vi "FindMaximum_MotorPower.vi"() -> ()   [LabVIEW 2017]
uses:
  <vilib>/myRIO/Instrument Drivers/Onboard IO/DIO/typedefs/DIO Reference.ctl
  <vilib>/myRIO/Common/Instrument Driver Framework/Utilities/typedefs/myRIO Generic Hardware Reference.ctl
  <vilib>/myRIO/Common/Instrument Driver Framework/Utilities/typedefs/Hardware Version Enum.ctl
  <vilib>/myRIO/Common/Instrument Driver Framework/Utilities/typedefs/myRIO v1.0 Reference.ctl
  <vilib>/myRIO/Common/Instrument Driver Framework/Utilities/typedefs/Generic FPGA Reference.ctl
  <vilib>/myRIO/Common/Instrument Driver Framework/myRIO v1.0/DIO/typedefs/DIO Channels List.ctl
  <vilib>/myRIO/Common/Instrument Driver Framework/myRIO v1.0/DIO/typedefs/DIO Channels Enum.ctl
  <vilib>/userdefined/High Color/nirio_resource_hc.ctl
  <vilib>/myRIO/Common/Instrument Driver Framework/Utilities/vis/Is FPGA Ref Available.vi
  <vilib>/myRIO/Common/Instrument Driver Framework/myRIO v1.0/DIO/vis/myRIO v1.1 Open DIO.vi
  <vilib>/myRIO/Instrument Drivers/Onboard IO/DIO/vis/Read.vi
  <vilib>/myRIO/Common/Instrument Driver Framework/Utilities/vis/Validate Channels.vi
  <vilib>/myRIO/Common/Instrument Driver Framework/myRIO v1.0/DIO/vis/myRIO v1.0 Reserve DIO.vi
  <vilib>/myRIO/Common/Instrument Driver Framework/myRIO v1.0/UART/vis/myRIO v1.0 Close UART.vi
  <vilib>/myRIO/Common/Instrument Driver Framework/myRIO v1.0/Resource Manager/vis/myRIO v1.0 Reserve Channel List.vi
  <vilib>/myRIO/Common/Instrument Driver Framework/myRIO v1.0/DIO/vis/myRIO v1.0 Build MUX Configuration DIO.vi
  <vilib>/myRIO/Common/Instrument Driver Framework/myRIO v1.0/Resource Manager/vis/myRIO v1.0 Reserve Channel.vi
  <vilib>/myRIO/Common/Instrument Driver Framework/myRIO v1.0/Resource Manager/vis/myRIO v1.0 Unreserve Channel.vi
  <vilib>/myRIO/Common/Instrument Driver Framework/myRIO v1.0/Resource Manager/vis/myRIO v1.0 Create Configuration List.vi
  <vilib>/myRIO/Common/Instrument Driver Framework/myRIO v1.0/Resource Manager/vis/myRIO v1.0 Build Mutex Name.vi
  <vilib>/Utility/VariantDataType/GetNumericInfo.vi
  <vilib>/Utility/error.llb/Error Cluster From Error Code.vi
  <vilib>/myRIO/Common/Instrument Driver Framework/myRIO v1.0/myRIO v1.1 Open.vi
  <vilib>/myRIO/Common/Instrument Driver Framework/Utilities/vis/IO Manager.vi
  <vilib>/myRIO/Common/Instrument Driver Framework/Utilities/vis/Configuration Manager.vi
  <vilib>/myRIO/Common/Instrument Driver Framework/myRIO v1.0/Resource Manager/vis/myRIO v1.0 Configure IO.vi
  <vilib>/myRIO/Common/Instrument Driver Framework/myRIO v1.0/myRIO v1.0 Close.vi
  <vilib>/myRIO/Common/Instrument Driver Framework/myRIO v1.0/DIO/vis/myRIO v1.0 Read DIO.vi
  <vilib>/myRIO/Common/Instrument Driver Framework/Utilities/vis/FPGA Ref Manager.vi
  <vilib>/myRIO/Common/Instrument Driver Framework/myRIO v1.0/myRIO v1.0 Reset FPGA.vi
  <vilib>/myRIO/Common/Instrument Driver Framework/myRIO v1.0/IRQ/vis/myRIO v1.0 IRQ Info FGV.vi
  <vilib>/myRIO/Common/Instrument Driver Framework/myRIO v1.0/IRQ/vis/myRIO v1.0 Timer IRQ Info FGV.vi
  <vilib>/myRIO/Common/Instrument Driver Framework/myRIO v1.0/IRQ/vis/myRIO v1.0 ISR Agent.vi
  <vilib>/myRIO/Express VI/Onboard Devices/Button/Button Express VI.xnode
  <vilib>/myRIO/Instrument Drivers/Onboard IO/DIO/vis/myRIO DIO Open.xnode
  <vilib>/myRIO/Instrument Drivers/Onboard IO/DIO/DIO.lvlib
  <vilib>/myRIO/Instrument Drivers/Utilities/Utilities.lvlib
panel:
  out "error out":errorcluster
  in  "milliseconds to wait":u32=3000
  in  "w2":i8(slide)=-100 scale=-100.0..100.0
  in  "w1":i8(slide)=-100 scale=-100.0..100.0
  in  "w3":i8(slide)=100 scale=-100.0..100.0
  in  "w4":i8(slide)=100 scale=-100.0..100.0
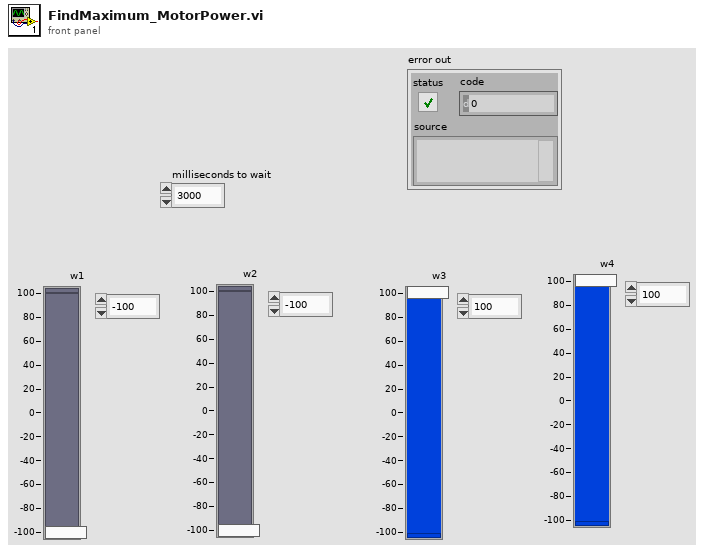
[diagram p1: front panel]
types:
  T1 = typedef "DIO.lvlib/DIO Reference.ctl" = cluster{"myRIO Reference":T2, "DIO Channels List":T6}
  T2 = typedef "myRIO Generic Hardware Reference.ctl" = cluster{"myRIO Model":T3, "myRIO Hardware Reference":T4}
  T3 = typedef "Hardware Version Enum.ctl" = enum16{"Unknown", "myRIO-1900", "myRIO-1950", "roboRIO", "NI ELVIS RIO CM"}
  T4 = typedef "myRIO v1.0 Reference.ctl" = cluster{"Generic FPGA Reference":T5, "Allow multiple opens":bool}
  T5 = typedef "Generic FPGA Reference.ctl" = refnum<k20>
  T6 = typedef "DIO Channels List.ctl" = T7[]
  T7 = typedef "DIO Channels Enum.ctl" = enum16{"Not Connected", "C/DIO0", "C/DIO1", "C/DIO2", "C/DIO3", "C/DIO4", "C/DIO5", "C/DIO6", "C/DIO7", "A/DIO0", "A/DIO1", "A/DIO2", "A/DIO3", "A/DIO4", "A/DIO5", "A/DIO6", "A/DIO7", "A/DIO8", "A/DIO9", "A/DIO10", "A/DIO11", "A/DIO12", "A/DIO13", "A/DIO14", "A/DIO15", "B/DIO0", "B/DIO1", "B/DIO2", "B/DIO3", "B/DIO4", "B/DIO5", "B/DIO6", "B/DIO7", "B/DIO8", "B/DIO9", "B/DIO10", "B/DIO11", "B/DIO12", "B/DIO13", "B/DIO14", "B/DIO15", "LED0", "LED1", "LED2", "LED3", "Button0", "DIO/DIO0", "DIO/DIO1", "DIO/DIO2", "DIO/DIO3", "DIO/DIO4", "DIO/DIO5", "DIO/DIO6", "DIO/DIO7", "DIO/DIO8", "DIO/DIO9", "SPI/CS0", "SPI/CS1", "SPI/CS2", "SPI/CS3", "LED RADIO (Green)", "LED RADIO (Red)", "LED COMM (Green)", "LED COMM (Red)", "LED MODE (Green)", "LED MODE (Red)"}
  T8 = typedef "nirio_resource_hc.ctl" = tag
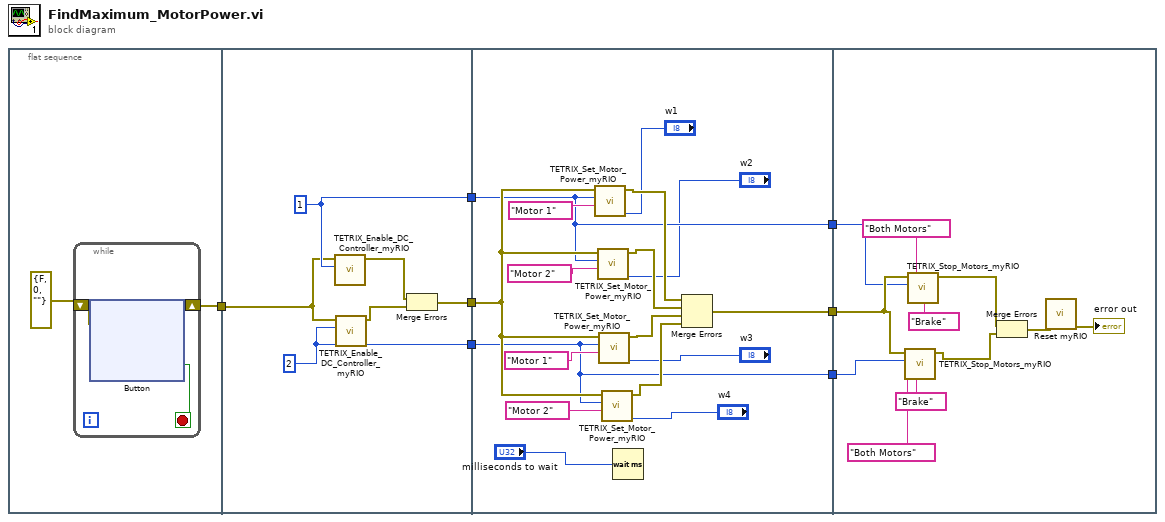
[diagram p0: block diagram]
diagram:
  n1 = flat-sequence {
    tunnel: [w9] -> w7
    tunnel: [w51] -> w6
    tunnel: [w50] -> w5
    tunnel: [w49] -> w4
    tunnel: w7 -> [w48]
    tunnel: w6 -> [w59]
    tunnel: w5 -> [w70]
    tunnel: w4 -> [w58]
    tunnel: [w61] -> w3
    tunnel: [w59] -> w2
    tunnel: [w58] -> w1
    tunnel: w3 -> [w81]
    tunnel: w2 -> [w80]
    tunnel: w1 -> [w79]
    frame #0 {
      n2 = while {
        shift-right: [w12] -> w9
        shift-left: errorcluster {"status"=FALSE, "code"=0, "source"=""} ("error constant") -> [w11]
        stop <- w10 stop-if-true
        n3 = xnode "Button"("error in (no error)"=w11) -> ("Value"=w10:bool, "error out"=w12:errorcluster)
      }
    }
    frame #1 {
      w49 = u8 2 ("Controller ID#  (I2C Address)")
      w51 = u8 1 ("Controller ID#  (I2C Address)")
      n4 = call <vilib>:"TETRIX_Enable_DC_Controller_myRIO.vi"("Controller ID#  (I2C Address)"=w51, "Error/Flow In"=w48) -> ("Error/Flow Out"=w53:errorcluster)  [unwired: 5 in]
      n5 = call <vilib>:"TETRIX_Enable_DC_Controller_myRIO.vi"("Controller ID#  (I2C Address)"=w49, "Error/Flow In"=w48) -> ("Error/Flow Out"=w52:errorcluster)  [unwired: 5 in]
      n6 = Merge Errors(w53, w52) -> (w50:errorcluster)
    }
    frame #2 {
      n7 = call <vilib>:"TETRIX_Set_Motor_Power_myRIO.vi"("Power (-100 to 100)  0 = Coast Stop  125 = Brake Stop"="w1", "Select Channel"="Motor 1", "Controller ID#  (I2C Address)"=w59, "Error/Flow In"=w70) -> ("Error/Flow Out"=w65:errorcluster)  [unwired: 3 in]
      n8 = call <vilib>:"TETRIX_Set_Motor_Power_myRIO.vi"("Power (-100 to 100)  0 = Coast Stop  125 = Brake Stop"="w2", "Select Channel"="Motor 2", "Controller ID#  (I2C Address)"=w59, "Error/Flow In"=w70) -> ("Error/Flow Out"=w64:errorcluster)  [unwired: 3 in]
      n9 = call <vilib>:"TETRIX_Set_Motor_Power_myRIO.vi"("Power (-100 to 100)  0 = Coast Stop  125 = Brake Stop"="w3", "Select Channel"="Motor 1", "Controller ID#  (I2C Address)"=w58, "Error/Flow In"=w70) -> ("Error/Flow Out"=w63:errorcluster)  [unwired: 3 in]
      n10 = call <vilib>:"TETRIX_Set_Motor_Power_myRIO.vi"("Power (-100 to 100)  0 = Coast Stop  125 = Brake Stop"="w4", "Select Channel"="Motor 2", "Controller ID#  (I2C Address)"=w58, "Error/Flow In"=w70) -> ("Error/Flow Out"=w62:errorcluster)  [unwired: 3 in]
      n11 = Wait (ms)(milliseconds to wait="milliseconds to wait") -> ()  [unwired: 1 out]
      n12 = Merge Errors(w65, w64, w63, w62) -> (w61:errorcluster)
    }
    frame #3 {
      n13 = call <vilib>:"TETRIX_Stop_Motors_myRIO.vi"("Stop Mode"="Brake", "Select Channel"="Both Motors", "Controller ID#  (I2C Address)"=w79, "Error/Flow In"=w81) -> ("Error/Flow Out"=w73:errorcluster)  [unwired: 3 in]
      n14 = call <vilib>:"TETRIX_Stop_Motors_myRIO.vi"("Stop Mode"="Brake", "Select Channel"="Both Motors", "Controller ID#  (I2C Address)"=w80, "Error/Flow In"=w81) -> ("Error/Flow Out"=w74:errorcluster)  [unwired: 3 in]
      n15 = Merge Errors(w74, w73) -> (w72:errorcluster)
      n16 = call <vilib>:"Reset myRIO.vi"("error in (no error)"=w72) -> ("error out"=→"error out":errorcluster)  [unwired: 10 in]
    }
  }
